vi "ATF-Add to List.vi"(10 "Enter Channel Name":string[](array[string]), 11 "Cluster in":T1) -> (2 "Boolean":bool, 3 "Cluster out":T1)   [LabVIEW 2022 SP3]
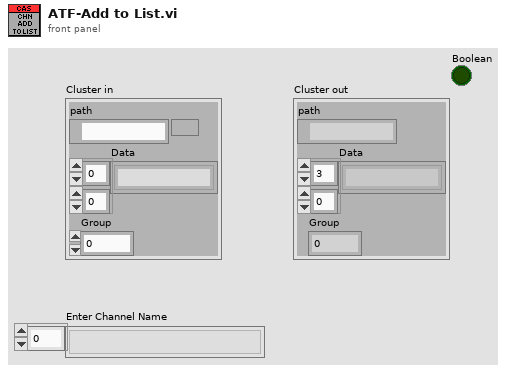
[diagram p1: front panel]
types:
  T1 = cluster{"path":path, "Data":string[][], "Group":i32}
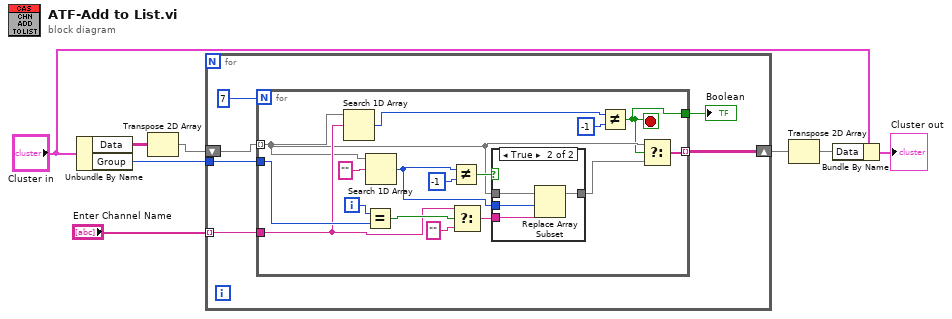
[diagram p0: block diagram]
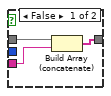
[diagram p2: hidden frame]
diagram:
  n1 = Unbundle By Name("Cluster in") -> ("Data"=w3:string[][], "Group"=w5:i32)
  n2 = Transpose 2D Array(2D array=w3) -> (transposed array=w8:string[][])
  n3 = for {
    tunnel: "Enter Channel Name" -> [w13] mode=indexing
    tunnel: w5 -> [w12]
    shift-right: [w11] -> w4
    shift-left: w8 -> [w14]
    n4 = for {
      N: 7 -> [_]
      tunnel: w12 -> [w27]
      tunnel: w13 -> [w19]
      tunnel: w14 -> [w18] mode=indexing
      tunnel: [w16] -> w11 mode=indexing
      tunnel: [w15] -> w9
      i -> [w28]
      stop <- w15 stop-if-true
      n5 = Search 1D Array(1D array=w18, element=w19) -> (index of element=w21:i32)  [unwired: 1 in]
      n6 = Equal?(x=w28, y=w27) -> (x = y?=w29:bool)
      n7 = Search 1D Array(1D array=w18, element="") -> (index of element=w22:i32)  [unwired: 1 in]
      n8 = Not Equal?(x=w22, y=-1) -> (x != y?=w23:bool)
      n9 = Select(t=w19, s=w29, f="") -> (s? t:f=w30:string)
      n10 = case shown="True" w23 {
        tunnel: w30 -> [w33 w36]
        tunnel: [w32 w35] -> w17
        tunnel: w18 -> [w31 w34]
        tunnel: w22 -> [_ w37]
        frame False {
          n11 = Build Array (concatenate)(w31, w33) -> (w32:string[])
        }
        frame True {
          n12 = Replace Array Subset(array=w34, new element=w36, index=w37) -> (w35:string[])
        }
      }
      n13 = Not Equal?(x=w21, y=-1) -> (x != y?=w15:bool)
      n14 = Select(t=w18, s=w15, f=w17) -> (s? t:f=w16:string[])
    }
    "Boolean" <- w9
  }
  n15 = Transpose 2D Array(2D array=w4) -> (transposed array=w7:string[][])
  n16 = Bundle By Name(cluster="Cluster in", "Data"=w7) -> (→"Cluster out":T1)
